vi "Format Attributes as Table.vi"(7 "Format for Real Values":string="%_3g", 8 "error in (no error)":errorcluster, 10 "Values":variant[](array[variant]), 11 "Names":string[](array[string])) -> (0 "error out":errorcluster, 3 "Formatted Table":string[][](array[string]))   [LabVIEW 2017]
doc: "Creates a 2D string table suitable for populating a table or multicolum listbox indicator."
panel:
  # "LVHDF5 Toolkit\nCopyright (c) 2005-2013 by Jason D. Sommerville\nCopyright (c) 2014 by UPVI, LLC.\n\nThis use and distribution of this file is governed by the terms found in \nLICENSE.txt distributed with this toolkit and installed at\n <user.lib>\\_lvhdf5\\LICENSE.txt"
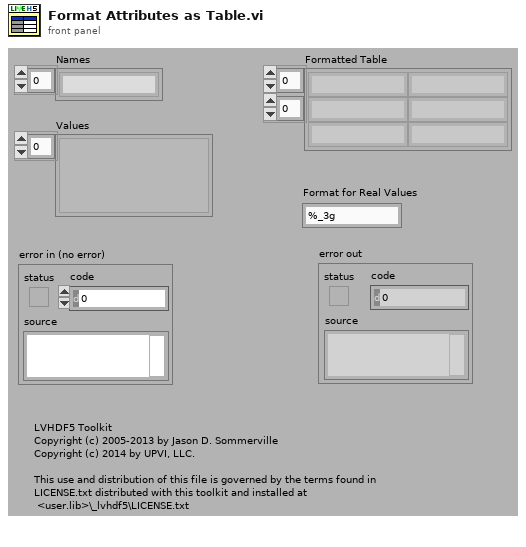
[diagram p1: front panel]
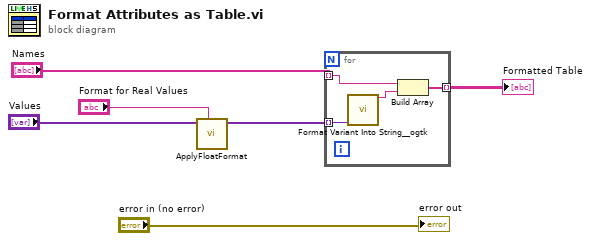
[diagram p0: block diagram]
diagram:
  n1 = call <vilib>:"ApplyFloatFormat.vi"("Format for Real Values"="Format for Real Values", "Values"="Values") -> ("Values Out"=w2:variant[])  [unwired: 7 in]
  n2 = for {
    tunnel: w2 -> [w10] mode=indexing
    tunnel: "Names" -> [w9] mode=indexing
    tunnel: [w7] -> w6 mode=indexing
    n3 = call <userlib>:"Format Variant Into String__ogtk.vi"("Variant"=w10) -> ("Output String"=w8:string)  [unwired: 13 in, 1 out]
    n4 = Build Array(w9, w8) -> (w7:string[])
  }
  "Formatted Table" <- w6
  "error out" <- "error in (no error)"
